vi "command to char.vi"(10 "Command":T1) -> (2 "char":string)   [LabVIEW 2017]
uses:
  typedefs/commandType.ctl
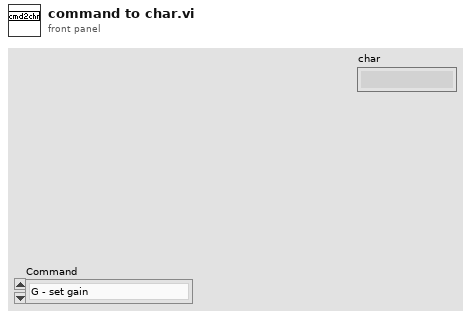
[diagram p1: front panel]
types:
  T1 = typedef "commandType.ctl" = enum16{"G - set gain", "C - activate coil", "D - deactivate coil", "L - set LED", "A - set AUTO", "V - set verbose", "T - set transmission", "R - get version", "Z - zero accelerometer"}
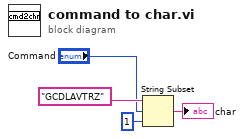
[diagram p0: block diagram]
diagram:
  n1 = String Subset(string="GCDLAVTRZ", offset (0)="Command", length (rest)=1 ("length (rest)")) -> (substring=→"char":string)
